vi "二维数组转一维（波形图.vi"(11 "二维数组":dbl[][](array[numeric])) -> (2 "第二列":dbl[](array[numeric]), 3 "第一列":dbl[](array[numeric]))   [LabVIEW 2015]
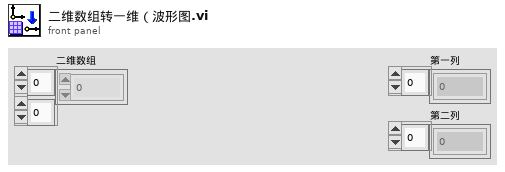
[diagram p1: front panel]
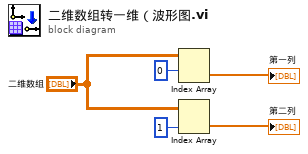
[diagram p0: block diagram]
diagram:
  n1 = Index Array(array="二维数组", index (row)=0) -> (element=→"第一列":dbl[])  [unwired: 1 in]
  n2 = Index Array(array="二维数组", index (row)=1 ("disabled index (col)")) -> (element=→"第二列":dbl[])  [unwired: 1 in]
